vi "IVCurveFit.vi"(11 "IVData":dbl[][](array[numeric])) -> (0 "error out":errorcluster, 1 "ChargeCapacitance":dbl, 2 "Conductance":dbl, 3 "Capacitance":dbl, 4 "bestFit":T1, 5 "residue":dbl, 6 "Fit":dbl[][](array[numeric]))   [LabVIEW 2020]
uses:
  <vilib>/Analysis/6fits.llb/Curve Fitting Criteria.ctl
  <vilib>/Utility/file.llb/Read Delimited Spreadsheet (DBL).vi
  <vilib>/gmath/NumericalOptimization/Nonlinear Curve Fit LM.vi
  <vilib>/gmath/NumericalOptimization/Nonlinear Curve Fit LM bound.vi
  <vilib>/Analysis/NI_AALPro.lvlib
  <vilib>/gmath/NI_Gmath.lvlib
panel:
  out "XY Graph 6":cluster{"IVData":dbl[], "IVData":dbl[]}(graph)
  out "number of function calls 2":i32
  out "number of function calls":i32
  out "best fit parameters 3":dbl[](array[numeric])
  out "XY Graph 5":cluster{dbl[], dbl[]}[](graph)
  out "error out 2":errorcluster
  out "appended array":dbl[](array[numeric])
  out "best fit parameters 2":dbl[](array[numeric])
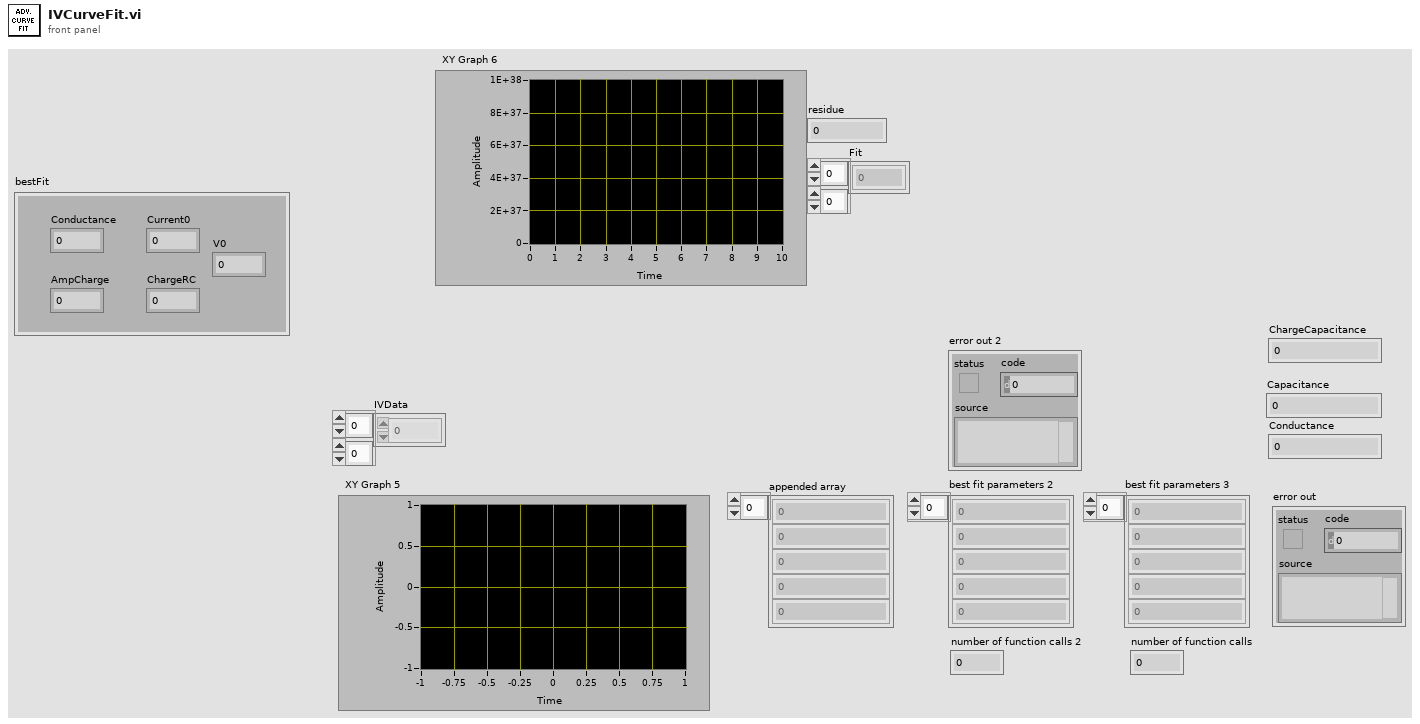
[diagram p1: front panel]
types:
  T1 = cluster{"Conductance":dbl, "Current0":dbl, "AmpCharge":dbl, "ChargeRC":dbl, "V0":dbl}
  T2 = cluster{"parameter minimum":dbl[], "parameter maximum":dbl[]}
  T3 = typedef "NI_AALPro.lvlib/Curve Fitting Criteria.ctl" = u16
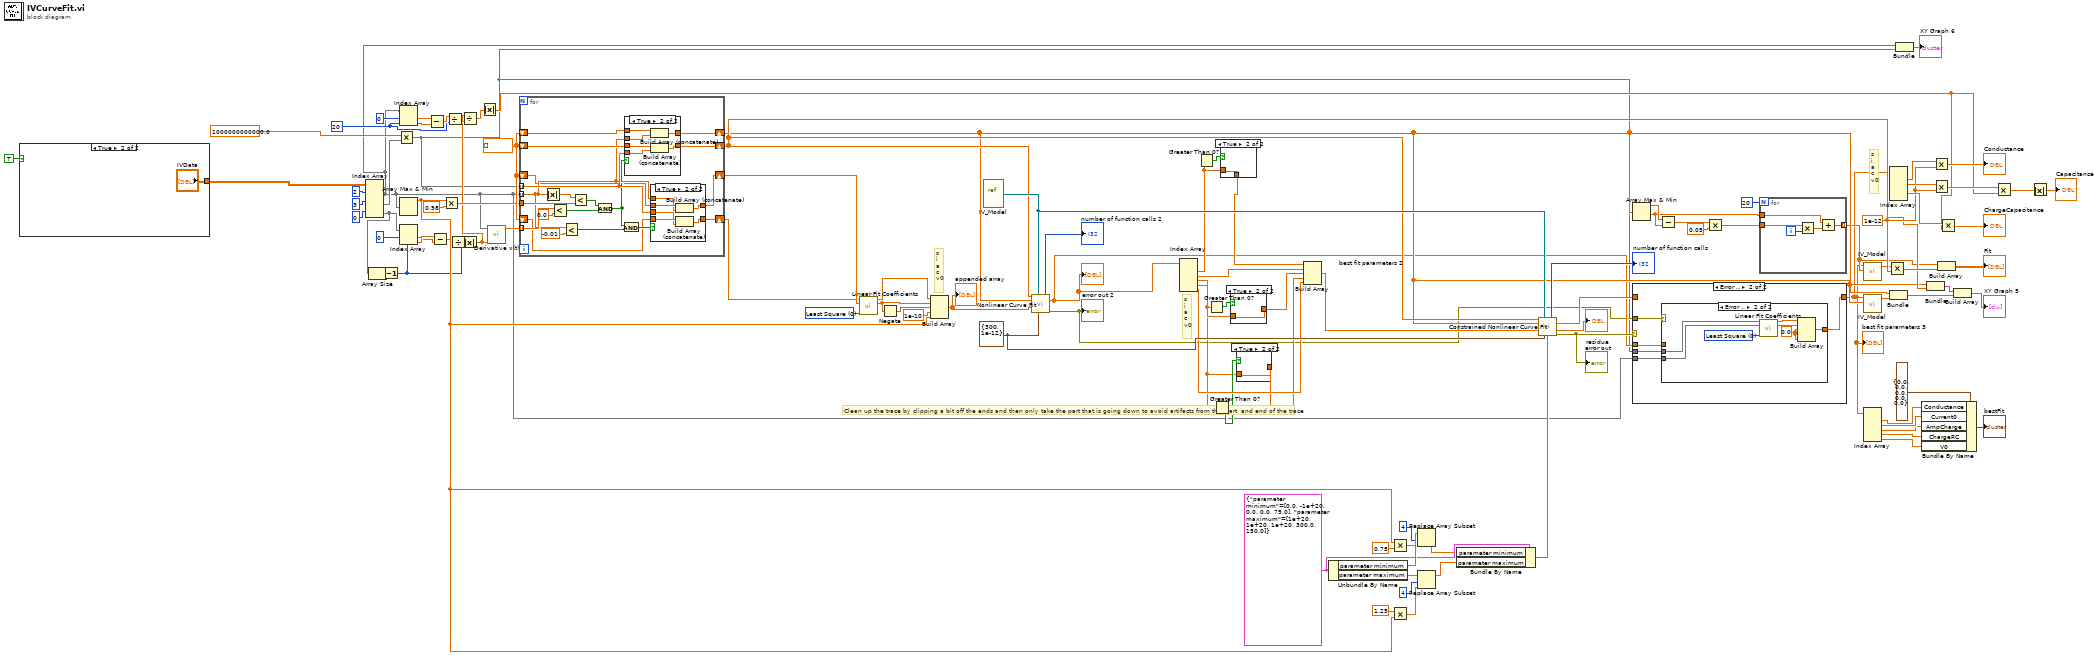
[diagram p0: block diagram]
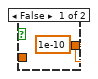
[diagram p4: hidden frame]
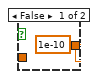
[diagram p5: hidden frame]
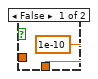
[diagram p6: hidden frame]
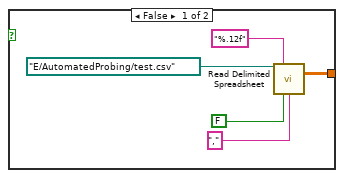
[diagram p7: hidden frame]
diagram:
  w25 = 1e-12
  w61 = T2 {"parameter minimum"=[0.0, -1e+20, 0.0, 0.0, 75.0], "parameter maximum"=[1e+20, 1e+20, 1e+20, 300.0, 150.0]} ("parameter bounds")
  w86 = cluster{"max iteration":i32, "tolerance":dbl} {"max iteration"=300, "tolerance"=1e-12} ("termination")
  w32 = 20 ("index")
  w103 = T3 0 items=["Least Square", "Least Absolute Residual", "Bisquare"] ("method")
  w104 = dbl[] []
  # "s\ni\na\nc\nv0"
  # "s\ni\na\nc\nv0"
  # "s\ni\na\nc\nv0"
  # "Clean up the trace by clipping a bit off the ends and then only take the part that is going down to avoid artifacts from the start  and end of the trace"
  n1 = case shown="True" TRUE {
    tunnel: [w107 "IVData"] -> w45
    frame False {
      n2 = call-poly <vilib>:"Read Delimited Spreadsheet.vi"("file path (dialog if empty)"=path "E:/AutomatedProbing/test.csv", "format (%.3f)"="%.12f", "transpose? (F)"=FALSE, "delimiter (\\t)"="," ("delimiter (\\t)")) -> ("all rows"=w107:dbl[][])  [unwired: 6 in, 5 out]
    }
    frame True {
    }
  }
  n3 = Index Array(array=w45, index (row) #1=2 ("index (row)"), index (row) #2=3 ("index (row)"), index (row) #3=0 ("index (row)")) -> (element #1=w2:dbl[], element #2=w29:dbl[], element #3=w40:dbl[])  [unwired: 3 in]
  n4 = Array Size(array=w40) -> (size(s)=w39:i32)
  n5 = Decrement(x=w39) -> (x-1=w38:i32)
  n6 = Multiply(x=1000000000000.0, y=w29) -> (x*y=w1:dbl[])
  n7 = Index Array(array=w2, index #1=0 ("index"), index #2=w32) -> (element #1=w101:dbl, element #2=w100:dbl)
  n8 = Array Max & Min(array=w2) -> (max value=w70:dbl)  [unwired: 3 out]
  n9 = Index Array(array=w40, index #1=0 ("index"), index #2=w38) -> (element #1=w36:dbl, element #2=w37:dbl)
  n10 = Subtract(x=w101, y=w100) -> (x-y=w33:dbl)
  n11 = Subtract(x=w37, y=w36) -> (x-y=w41:dbl)
  n12 = Multiply(x=w70, y=0.98) -> (x*y=w102:dbl)
  n13 = Divide(x=w33, y=w32) -> (x/y=w34:dbl)
  n14 = Divide(x=w41, y=w38) -> (x/y=w35:dbl)
  n15 = Absolute Value(x=w35) -> (abs(x)=w31:dbl)
  n16 = Divide(x=w31, y=w34) -> (x/y=w50:dbl)
  n17 = Absolute Value(x=w50) -> (abs(x)=w49:dbl)
  n18 = call <vilib>:"Derivative x(t).vi"("dt"=w31, "X"=w2) -> ("dX/dt"=w105:dbl[])  [unwired: 8 in, 1 out]
  n19 = for {
    tunnel: w102 -> [w129]
    tunnel: w2 -> [w119] mode=indexing
    tunnel: w1 -> [w120] mode=indexing
    shift-right: [w132] -> w23
    shift-left: w104 -> [w122]
    shift-right: [w131] -> w24
    shift-left: w104 -> [w121]
    tunnel: w105 -> [w127] mode=indexing
    shift-right: [w124] -> w96
    shift-left: w104 -> [w114]
    shift-right: [w123] -> w95
    shift-left: w104 -> [w113]
    n20 = Absolute Value(x=w119) -> (abs(x)=w130:dbl)
    n21 = Less?(x=w127, y=0.0) -> (x < y?=w125:bool)
    n22 = Less?(x=w119, y=-0.01) -> (x < y?=w116:bool)
    n23 = Less?(x=w130, y=w129) -> (x < y?=w128:bool)
    n24 = And(x=w128, y=w125) -> (x .and. y?=w117:bool)
    n25 = And(x=w117, y=w116) -> (x .and. y?=w115:bool)
    n26 = case shown="True" w117 {
      tunnel: w122 -> [w142 w148]
      tunnel: w121 -> [w141 w147]
      tunnel: [w142 w146] -> w132
      tunnel: [w141 w145] -> w131
      tunnel: w119 -> [_ w144]
      tunnel: w120 -> [_ w143]
      frame False {
      }
      frame True {
        n27 = Build Array (concatenate)(w148, w144) -> (w146:dbl[])
        n28 = Build Array (concatenate)(w147, w143) -> (w145:dbl[])
      }
    }
    n29 = case shown="True" w115 {
      tunnel: w114 -> [w134 w140]
      tunnel: w113 -> [w133 w139]
      tunnel: [w134 w138] -> w124
      tunnel: [w133 w137] -> w123
      tunnel: w119 -> [_ w136]
      tunnel: w120 -> [_ w135]
      frame False {
      }
      frame True {
        n30 = Build Array (concatenate)(w140, w136) -> (w138:dbl[])
        n31 = Build Array (concatenate)(w139, w135) -> (w137:dbl[])
      }
    }
  }
  n32 = call <vilib>:"Linear Fit Coefficients.vi"("Y"=w95, "X"=w96, "method"=w103) -> ("slope"=w94:dbl, "intercept"=w92:dbl)  [unwired: 10 in, 1 out]
  n33 = Negate(x=w92) -> (-x=w91:dbl)
  n34 = Build Array(w94, w92, w91, 1e-10 ("element"), w70) -> (w84:dbl[])
  "appended array" <- w84
  n35 = vi-ref "IV_Model.vi"() -> (w87:refnum<vi>)
  n36 = call-poly <vilib>:"Nonlinear Curve Fit.vi"("Y"=w24, "f(x,a)"=w87, "X"=w23, "initial parameters"=w84, "termination"=w86) -> ("number of function calls"=→"number of function calls 2":i32, "best fit parameters"=w4:dbl[], "error out"=w3:errorcluster)  [unwired: 5 in, 3 out]
  "best fit parameters 2" <- w4
  "error out 2" <- w3
  n37 = Index Array(array=w4) -> (element #1=w79:dbl, element #2=w77:dbl, element #3=w75:dbl, element #4=w72:dbl, element #5=w81:dbl)  [unwired: 5 in]
  n38 = Greater Than 0?(x=w79) -> (x > 0?=w80:bool)
  n39 = Greater Than 0?(x=w75) -> (x > 0?=w76:bool)
  n40 = Greater Than 0?(x=w72) -> (x > 0?=w73:bool)
  n41 = case shown="True" w80 {
    tunnel: w79 -> [_ w150]
    tunnel: [1e-10 ("element") w150] -> w78
    frame False {
    }
    frame True {
    }
  }
  n42 = case shown="True" w76 {
    tunnel: w75 -> [_ w152]
    tunnel: [1e-10 ("element") w152] -> w74
    frame False {
    }
    frame True {
    }
  }
  n43 = case shown="True" w73 {
    tunnel: w72 -> [_ w154]
    tunnel: [1e-10 ("element") w154] -> w71
    frame False {
    }
    frame True {
    }
  }
  n44 = Build Array(w78, w77, w74, w71, w81) -> (w57:dbl[])
  n45 = Unbundle By Name(w61) -> ("parameter minimum"=w67:dbl[], "parameter maximum"=w63:dbl[])
  n46 = Multiply(x=w70, y=0.75) -> (x*y=w65:dbl)
  n47 = Multiply(x=1.25, y=w70) -> (x*y=w62:dbl)
  n48 = Replace Array Subset(array=w67, new element=w65, index=4) -> (w59:dbl[])
  n49 = Replace Array Subset(array=w63, new element=w62, index=4) -> (w58:dbl[])
  n50 = Bundle By Name(cluster=w61, "parameter minimum"=w59, "parameter maximum"=w58) -> (w60:T2)
  n51 = call-poly <vilib>:"Constrained Nonlinear Curve Fit.vi"("Y"=w24, "f(x,a)"=w87, "X"=w23, "initial parameters"=w57, "termination"=w86, "parameter bounds"=w60) -> ("number of function calls"=→"number of function calls":i32, "best fit parameters"=w6:dbl[], "residue"=→"residue":dbl, "error out"=w7:errorcluster)  [unwired: 4 in, 2 out]
  "error out" <- w7
  n52 = Array Max & Min(array=w23) -> (max value=w22:dbl, min value=w20:dbl)  [unwired: 2 out]
  n53 = case shown="Error .." w7 {
    tunnel: w6 -> [w155 _]
    tunnel: [w155 w159] -> w5
    tunnel: w4 -> [_ w158]
    tunnel: w3 -> [_ w160]
    tunnel: w2 -> [_ w157]
    tunnel: w1 -> [_ w156]
    frame No Error {
    }
    frame Error {
      n54 = case shown="Error .." w160 {
        tunnel: [w161 w162] -> w159
        tunnel: w158 -> [w161 _]
        tunnel: w157 -> [_ w167]
        tunnel: w156 -> [_ w166]
        frame No Error {
        }
        frame Error {
          w165 = 0.0 ("element")
          w168 = T3 0 items=["Least Square", "Least Absolute Residual", "Bisquare"] ("method")
          n55 = call <vilib>:"Linear Fit Coefficients.vi"("Y"=w166, "X"=w167, "method"=w168) -> ("slope"=w164:dbl, "intercept"=w163:dbl)  [unwired: 10 in, 1 out]
          n56 = Build Array(w164, w163, w165, w165, w165) -> (w162:dbl[])
        }
      }
    }
  }
  "best fit parameters 3" <- w5
  n57 = Subtract(x=w22, y=w20) -> (x-y=w19:dbl)
  n58 = Multiply(x=w19, y=0.05) -> (x*y=w16:dbl)
  n59 = for {
    N: 20 -> [_]
    tunnel: w20 -> [w173]
    tunnel: w16 -> [w171]
    tunnel: [w169] -> w17 mode=indexing
    i -> [w170]
    n60 = Multiply(x=w171, y=w170) -> (x*y=w172:dbl)
    n61 = Add(x=w173, y=w172) -> (x+y=w169:dbl)
  }
  n62 = call "IV_Model.vi"("X"=w17, "a"=w5) -> ("f(X,a)"=w18:dbl[])  [unwired: 2 in, 2 out]
  n63 = call "IV_Model.vi"("X"=w23, "a"=w5) -> ("f(X,a)"=w88:dbl[])  [unwired: 2 in, 2 out]
  n64 = Index Array(array=w5) -> (element #1=w12:dbl, element #2=w11:dbl, element #3=w10:dbl, element #4=w9:dbl, element #5=w8:dbl)  [unwired: 5 in]
  n65 = Multiply(x=w18, y=w25) -> (x*y=w26:dbl[])
  n66 = Index Array(array=w5) -> (element #1=w56:dbl, element #2=w55:dbl, element #4=w52:dbl)  [unwired: 5 in, 2 out]
  n67 = Bundle(w23, "f(X,a)"=w88) -> (w89:cluster{dbl[], "f(X,a)":dbl[]})  [unwired: 1 in]
  n68 = Bundle("IVData"=w2, w1) -> (→"XY Graph 6":cluster{"IVData":dbl[], dbl[]})  [unwired: 1 in]
  n69 = Bundle By Name(cluster=T1 {"Conductance"=0.0, "Current0"=0.0, "AmpCharge"=0.0, "ChargeRC"=0.0, "V0"=0.0} ("bestFit"), "Conductance"=w12, "Current0"=w11, "AmpCharge"=w10, "ChargeRC"=w9, "V0"=w8) -> (→"bestFit":T1)
  n70 = Bundle(w23, w24) -> (w85:cluster{dbl[], dbl[]})  [unwired: 1 in]
  n71 = Multiply(x=w56, y=w25) -> (x*y=→"Conductance":dbl)
  n72 = Multiply(x=w55, y=w25) -> (x*y=w54:dbl)
  n73 = Build Array(w17, w26) -> (→"Fit":dbl[][])
  n74 = Multiply(x=w52, y=w49) -> (x*y=→"ChargeCapacitance":dbl)
  n75 = Build Array(w85, w89) -> (→"XY Graph 5":cluster{dbl[], "f(X,a)":dbl[]}[])
  n76 = Multiply(x=w54, y=w49) -> (x*y=w99:dbl)
  n77 = Absolute Value(x=w99) -> (abs(x)=→"Capacitance":dbl)
